vi "Create User Event - Stop.vi"(8 "error in (no error)":errorcluster, 10 "VI in":refnum<vi>) -> (0 "error out":errorcluster, 2 "Event Registration Refnum":refnum<event-registration>, 3 "User Event":refnum<user-event>)   [LabVIEW 2020, in "User Event - Stop.lvlib"]
doc: "Create a boolean user event that will be used to stop the event loop from the message handling loop."
uses:
  User Event - Stop.lvlib
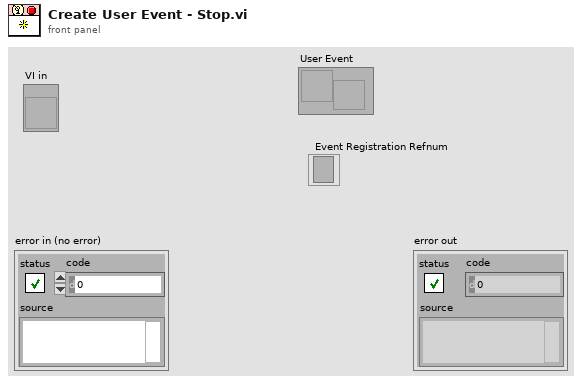
[diagram p1: front panel]
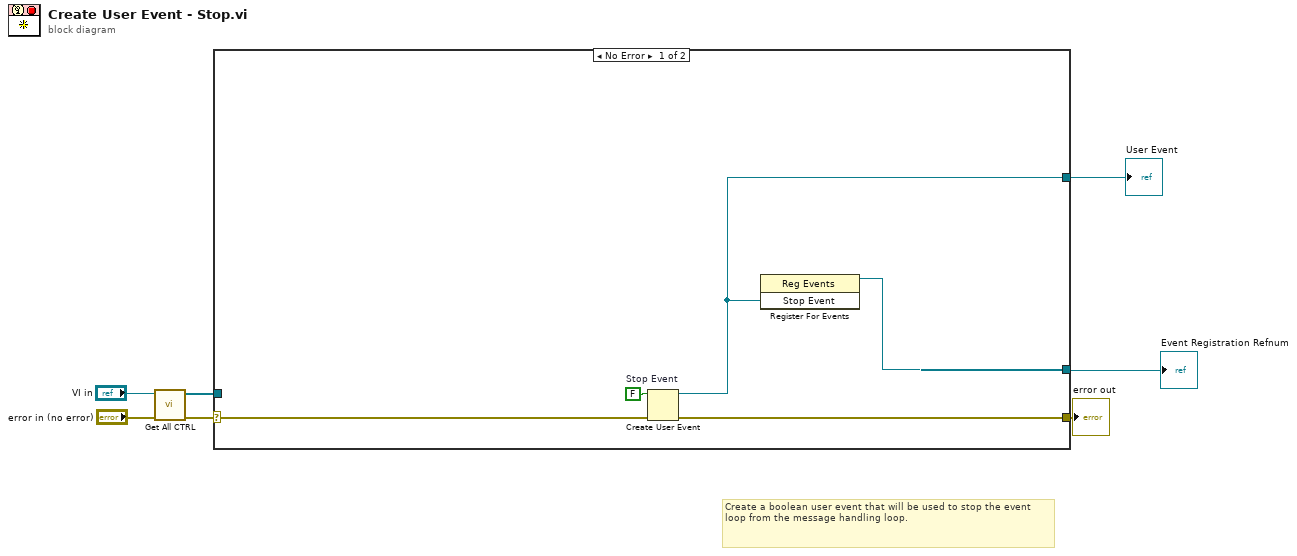
[diagram p0: block diagram]
diagram:
  # "Create a boolean user event that will be used to stop the event loop from the message handling loop."
  n1 = call "Get All CTRL.vi"("error in (no error)"="error in (no error)", "This VI"="VI in") -> ("error out"=w3:errorcluster, "CTRL REF"=w1:refnum<vi>[])  [unwired: 8 in]
  n2 = case shown="No Error" w3 {
    selector: w3 -> [w10 w13]
    tunnel: [w9 _] -> w7
    tunnel: [w11 w13] -> w6
    tunnel: [w8 _] -> w5
    tunnel: w1 -> [_ _]
    frame No Error {
      w12 = FALSE  # Stop Event
      n3 = Create User Event(user event datatype=w12, error in=w10) -> (user event=w9:refnum<user-event>, error out=w11:errorcluster)
      n4 = register-events(w9) -> (reference out=w8:refnum<event-registration>)  [unwired: 2 in, 1 out]
    }
    frame Error {
    }
  }
  "User Event" <- w7
  "error out" <- w6
  "Event Registration Refnum" <- w5
